vi "Edit Configuration.vi"(8 "error in (no error)":errorcluster, 9 "Edit Configuration Actions":T1=enum."Update", 10 "Data Type Object":refnum<class "Generic Data Type.lvclass">, 11 "DataGrid Config in":refnum<class "DataGrid Config.lvclass">) -> (0 "error out":errorcluster, 3 "DataGrid Config out":refnum<class "DataGrid Config.lvclass">)   [LabVIEW 2018, in "DataGrid Config.lvclass"]
uses:
  DataGrid Config.lvclass
  Edit Configuration Actions.ctl
  Data Type Classes/Generic/Generic Data Type.lvclass
  DataGrid Config.lvclass/DataGrid Config.ctl
  Data Type Classes/Generic/Generic Data Type.lvclass/Generic Data Type.ctl
  Data Type Classes/Generic/Read Column Index.vi
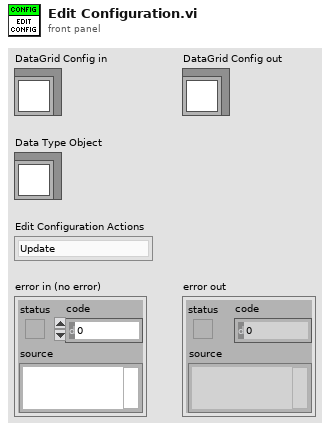
[diagram p1: front panel]
types:
  T1 = typedef "DataGrid Config.lvclass/Edit Configuration Actions.ctl" = enum16{"Add", "Remove", "Update", "Move Up", "Move Down"}
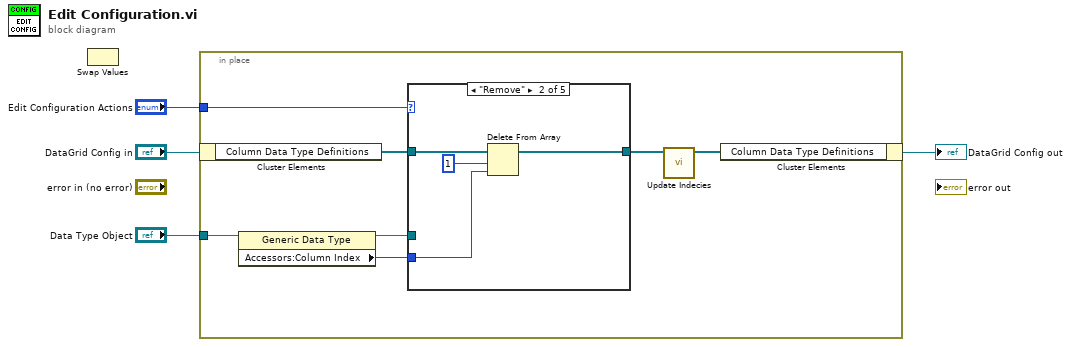
[diagram p0: block diagram]
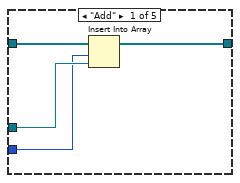
[diagram p2: hidden frame]
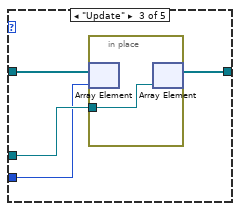
[diagram p3: hidden frame]
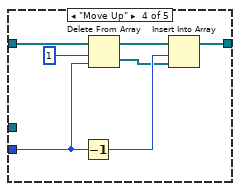
[diagram p4: hidden frame]
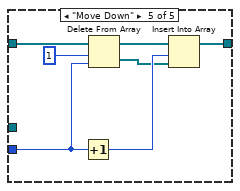
[diagram p5: hidden frame]
diagram:
  n1 = Swap Values() -> ()  [unwired: 3 in, 2 out]
  n2 = in-place {
    in-place-border: "Edit Configuration Actions" -> [w11]
    in-place-border: "Data Type Object" -> [w9]
    n3 = in-place-cluster #1("DataGrid Config in") -> ("Column Data Type Definitions"=w10:refnum<class "Generic Data Type.lvclass">[])
    n4 = property class="Generic Data Type"(reference=w9) -> (reference out=w6:refnum<class "Generic Data Type.lvclass">, "Accessors:Column Index"=w5:i32)  [unwired: 1 in, 1 out]
    n5 = case shown="\"Remove\"" w11 {
      tunnel: w10 -> [w15 w19 w23 w28 w35]
      tunnel: w6 -> [w14 _ w21 _ _]
      tunnel: [w13 w18 w22 w27 w32] -> w7
      tunnel: w5 -> [w12 w16 w20 w26 w34]
      frame "Add" {
        n6 = Insert Into Array(array=w15, index=w12, new element=w14) -> (w13:refnum<class "Generic Data Type.lvclass">[])
      }
      frame "Remove" {
        n7 = Delete From Array(array=w19, length=1, index=w16) -> (array with subset deleted=w18:refnum<class "Generic Data Type.lvclass">[])  [unwired: 1 out]
      }
      frame "Update" {
        n8 = in-place {
          in-place-border: w21 -> [w24]
          n9 = in-place-array #2(w23, w20) -> ()  [unwired: 1 out]
          n10 = in-place-array #2(w24) -> (w22:refnum<class "Generic Data Type.lvclass">[])  [unwired: 1 out]
        }
      }
      frame "Move Up" {
        n11 = Decrement(x=w26) -> (x-1=w31:i32)
        n12 = Delete From Array(array=w28, length=1, index=w26) -> (deleted portion=w30:refnum<class "Generic Data Type.lvclass">[], array with subset deleted=w29:refnum<class "Generic Data Type.lvclass">[])
        n13 = Insert Into Array(array=w29, index=w31, new element=w30) -> (w27:refnum<class "Generic Data Type.lvclass">[])
      }
      frame "Move Down" {
        n14 = Increment(x=w34) -> (x+1=w38:i32)
        n15 = Delete From Array(array=w35, length=1, index=w34) -> (deleted portion=w37:refnum<class "Generic Data Type.lvclass">[], array with subset deleted=w36:refnum<class "Generic Data Type.lvclass">[])
        n16 = Insert Into Array(array=w36, index=w38, new element=w37) -> (w32:refnum<class "Generic Data Type.lvclass">[])
      }
    }
    n17 = call "Update Indecies.vi"("Column Data Type Definitions in"=w7) -> ("Column Data Type Definitions out"=w8:refnum<class "Generic Data Type.lvclass">[])  [unwired: 9 in, 1 out]
    n18 = in-place-cluster #1("Column Data Type Definitions"=w8) -> (→"DataGrid Config out":refnum<class "DataGrid Config.lvclass">)
  }
